vi "AK RS-xxx Factory Wrapper.vi"(8 "error in (no error)":errorcluster, 10 "AK RS-xxx Settings":T1 caption="AK RS-xxx settings") -> (0 "error out":errorcluster, 3 "AK RS-xxx out":refnum<class "AK RS-xxx.lvclass">)   [LabVIEW 2018, in "Instrument Addon Scripting API.lvlib"]
doc: "Instantiates a new AK RS-xxx Protocol object using the provided AK RS-xxx settings."
uses:
  Instrument Addon Scripting API.lvlib
  Addon/Support Libraries/Protocols.lvlibp/AK RS-xxx/AK RS-xxx Settings.ctl
  Addon/Support Libraries/Protocols.lvlibp/AK RS-xxx/AK RS-xxx.lvclass
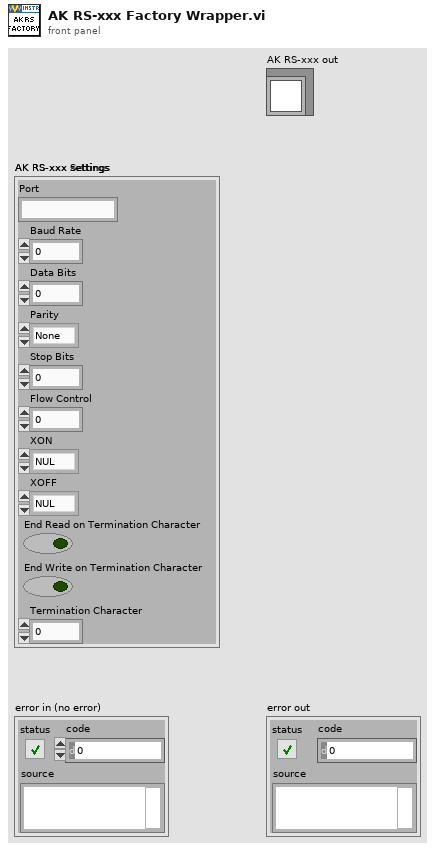
[diagram p1: front panel]
types:
  T1 = typedef "Protocols.lvlibp/AK RS-xxx.lvclass/AK RS-xxx Settings.ctl" = cluster{"Port":string, "Baud Rate":u32, "Data Bits":u16, "Parity":enum16{"None", "Odd", "Even", "Mark", "Space"}, "Stop Bits":u16, "Flow Control":u16, "XON":enum16{"NUL", "SOH", "STX", "ETX", "EOT", "ENQ", "ACK", "BEL", "BS", "HT", "LF", "VT", "FF", "CR", "SO", "SI", "DLE", "DC1", "DC2", "DC3", "DC4", "NAK", "SYN", "ETB", "CAN", "EM", "SUB", "ESC", "FS", "GS", "RS", "US", "SP", "!", "\"", "#", "$", "%", "&", "'", "(", ")", "*", "+", ",", "- (-)", ".", "/", "0", "1", "2", "3", "4", "5", "6", "7", "8", "9", ":", ";", "<", "=", ">", "?", "@", "A", "B", "C", "D", "E", "F", "G", "H", "I", "J", "K", "L", "M", "N", "O", "P", "Q", "R", "S", "T", "U", "V", "W", "X", "Y", "Z", "[", "\\", "]", "^", "_", "`", "a", "b", "c", "d", "e", "f", "g", "h", "i", "j", "k", "l", "m", "n", "o", "p", "q", "r", "s", "t", "u", "v", "w", "x", "y", "z", "{", "|", "}", "~"}, "XOFF":enum16{"NUL", "SOH", "STX", "ETX", "EOT", "ENQ", "ACK", "BEL", "BS", "HT", "LF", "VT", "FF", "CR", "SO", "SI", "DLE", "DC1", "DC2", "DC3", "DC4", "NAK", "SYN", "ETB", "CAN", "EM", "SUB", "ESC", "FS", "GS", "RS", "US", "SP", "!", "\"", "#", "$", "%", "&", "'", "(", ")", "*", "+", ",", "- (-)", ".", "/", "0", "1", "2", "3", "4", "5", "6", "7", "8", "9", ":", ";", "<", "=", ">", "?", "@", "A", "B", "C", "D", "E", "F", "G", "H", "I", "J", "K", "L", "M", "N", "O", "P", "Q", "R", "S", "T", "U", "V", "W", "X", "Y", "Z", "[", "\\", "]", "^", "_", "`", "a", "b", "c", "d", "e", "f", "g", "h", "i", "j", "k", "l", "m", "n", "o", "p", "q", "r", "s", "t", "u", "v", "w", "x", "y", "z", "{", "|", "}", "~"}, "End Read on Termination Character":bool, "End Write on Termination Character":bool, "Termination Character":u8}
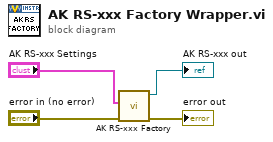
[diagram p0: block diagram]
diagram:
  n1 = call "AK RS-xxx Factory.vi"("Error In"="error in (no error)", "AK RS-xxx Settings"="AK RS-xxx Settings") -> ("Error Out"=→"error out":errorcluster, "AK RS-xxx Out"=→"AK RS-xxx out":refnum<class "AK RS-xxx.lvclass">)  [unwired: 8 in]
